vi "NewController.vi"(6 "Database":refnum<class "Database.lvclass">, 8 "error in (no error)":errorcluster, 9 "Name('')":string, 10 "ID(\"\")":string, 11 "Member_Actor in":refnum<class "Member_Actor.lvclass">) -> (0 "error out":errorcluster, 3 "Member_Actor out":refnum<class "Member_Actor.lvclass">)   [LabVIEW 2015, in "Member_Actor.lvlib" / "Member_Actor.lvclass"]
uses:
  Member_Actor.lvclass
  API/_Database/Database.lvclass
  Member_Actor.lvclass/Member_Actor.ctl
  Admin_Actor/Setting/g_setting.vi
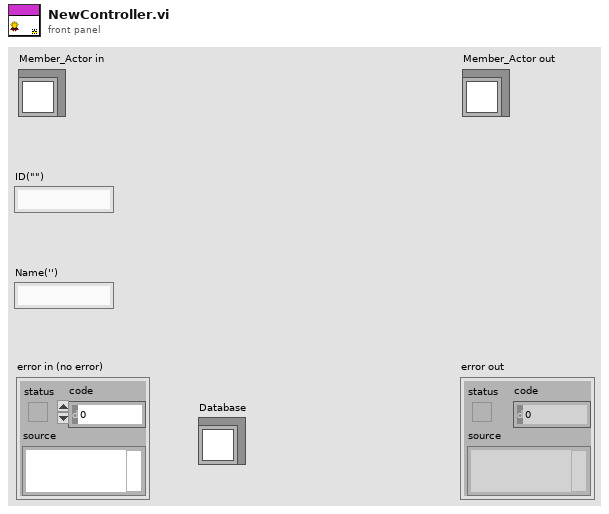
[diagram p1: front panel]
types:
  T1 = typedef "LVDateTimeRec.ctl" = cluster{"fractional second":dbl, "second":i32, "minute":i32, "hour":i32, "day of month":i32, "month":i32, "year":i32, "day of week":i32, "day of year":i32, "DST":i32}
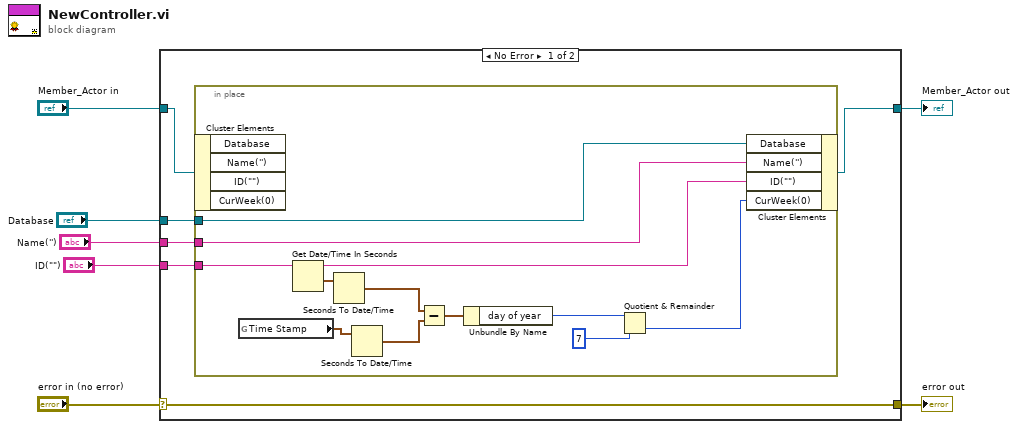
[diagram p0: block diagram]
diagram:
  n1 = case shown="No Error" "error in (no error)" {
    selector: "error in (no error)" -> [w13 w26]
    tunnel: [w13 w26] -> w6
    tunnel: [w8 w25] -> w4
    tunnel: "Member_Actor in" -> [w12 w25]
    tunnel: "ID(\"\")" -> [w11 _]
    tunnel: "Name('')" -> [w10 _]
    tunnel: "Database" -> [w9 _]
    frame No Error {
      n2 = in-place {
        in-place-border: w11 -> [w22]
        in-place-border: w10 -> [w21]
        in-place-border: w9 -> [w20]
        n3 = in-place-cluster #1(w12) -> ()  [unwired: 4 out]
        n4 = global read "g_setting.vi" "Time Stamp"() -> (w23:timestamp)
        n5 = Get Date/Time In Seconds() -> (seconds since 1Jan1904=w24:timestamp)
        n6 = Seconds To Date/Time(time stamp (now)=w24) -> (date time rec=w19:T1)  [unwired: 1 in]
        n7 = Seconds To Date/Time(time stamp (now)=w23) -> (date time rec=w17:T1)  [unwired: 1 in]
        n8 = Subtract(x=w19, y=w17) -> (x-y=w18:T1)
        n9 = Unbundle By Name(w18) -> ("day of year"=w16:i32)
        n10 = Quotient & Remainder(x=w16, y=7) -> (floor(x/y)=w14:i32)  [unwired: 1 out]
        n11 = in-place-cluster #1("Database"=w20, "Name('')"=w21, "ID(\"\")"=w22, "CurWeek(0)"=w14) -> (w8:refnum<class "Member_Actor.lvclass">)
      }
    }
    frame Error {
    }
  }
  "error out" <- w6
  "Member_Actor out" <- w4
